vi "Main.vi"(11 "Module Admin":refnum<class "Delacor_lib_QMH_Module Admin.lvclass">) -> ()   [LabVIEW 2024, in "Handheld Scanner.lvlib"]
doc: "This template is based off of the Queued Message Handler design pattern and the Queued Message Handler project template that ships with LabVIEW.\n\nThe main difference is that the queue is private to this module and communication between modules is performed via Broadcast and Request events.\n\nRequest events are wrapped in public API methods and are handled in the Event Handling Loop (EHL) of this VI. Any module can register for Broadcast events sent by this module. The EHL generates messages based on user interface actions.\n\nThe Message Handling Loop (MHL) processes messages generated by the EHL, or by other messages. The messages are string values, so new messages can be added easily to the Message Cases case structure in the MHL. Each message cluster can also provide an optional value for Message Data, which is a variant that can be converted to whatever message-specific data is required.\n_____\nBased on DQMH Dev Tools: Project Template 7.1.0.1503."
uses:
  Handheld Scanner.lvlib
  <vilib>/Delacor/Delacor QMH/Libraries/Module Admin_class/Delacor_lib_QMH_Module Admin.lvclass
  Module Data--cluster.ctl
  <vilib>/Delacor/Delacor QMH/Libraries/Message Queue_class/Delacor_lib_QMH_Message Queue.lvclass/Delacor_lib_QMH_Message Queue.ctl
  Stop Argument--cluster.ctl
  <vilib>/Delacor/Delacor QMH/Libraries/Module Admin_class/Delacor_lib_QMH_Module Admin.lvclass/Delacor_lib_QMH_Module Admin.ctl
  connect Argument--cluster.ctl
  read data Argument--cluster.ctl
  <vilib>/Utility/miscctls.llb/LVPointTypeDef.ctl
  GUI/Controls/HW Modules.ctl
  <vilib>/Delacor/Delacor QMH/Libraries/Message Queue_class/Delacor_lib_QMH_Enqueue Message (Single).vi
  <vilib>/Delacor/Delacor QMH/Libraries/Module Admin_class/Delacor_lib_QMH_Get External Launch.vi
  <vilib>/Delacor/Delacor QMH/Libraries/Message Queue_class/Delacor_lib_QMH_Message Queue.lvclass
  Controller/Controller.lvlib
panel:
  out "error out":errorcluster
  out "Status":string
  in  "Simulate MHL Error":bool
  in  "Simulate EHL Error":bool
  # "Other processes communicate with this Module via its Public API (wrappers for its Request Events).\n\nThis Module communicates with other processes via its Broadcast Events.\nAny process that wants to receive these messages can register for this module's Broadcast events."
  # "This template is for the DQMH framework. See the block diagram for more information on how to use this template."
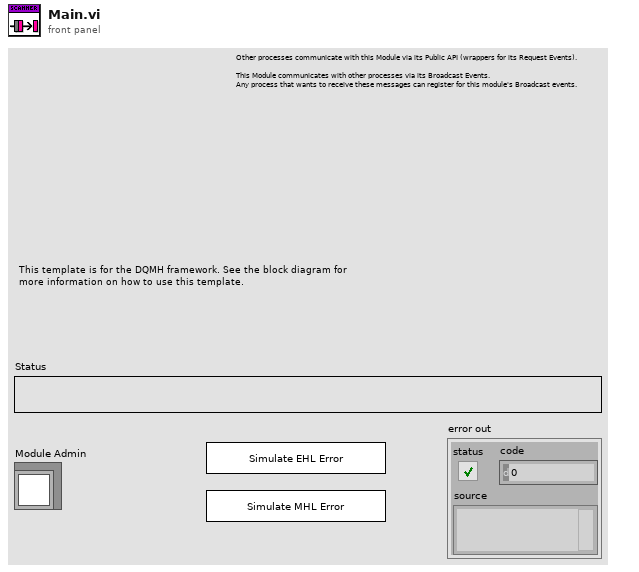
[diagram p1: front panel]
types:
  T1 = typedef "Handheld Scanner.lvlib/Request Events--cluster.ctl" = cluster{"Stop Module":refnum<user-event>, "Show Panel":refnum<user-event>, "Hide Panel":refnum<user-event>, "Get Module Execution Status":refnum<user-event>, "Show Diagram":refnum<user-event>, "connect":refnum<user-event>, "Private.read data":refnum<user-event>}
  T2 = typedef "Handheld Scanner.lvlib/Module Data--cluster.ctl" = cluster{"Status":string}
  T3 = enum32{"invalid lock state", "Not Locked", "Locked (No Password)", "Password-protected"}
  T4 = typedef "Handheld Scanner.lvlib/Stop Argument--cluster.ctl" = cluster{"Origin":string, "Exit via Stop Module Req?":bool, "Wait for Module to stop?":bool}
  T5 = typedef "Handheld Scanner.lvlib/connect Argument--cluster.ctl" = cluster{"VISA":refnum<visa-resource-name>}
  T6 = typedef "Handheld Scanner.lvlib/read data Argument--cluster.ctl" = cluster{"Boolean":bool}
  T7 = typedef "LVPointTypeDef.ctl" = cluster{"Horizontal":i16, "Vertical":i16}
  T8 = enum32{"Invalid", "Standard", "Closed", "Hidden", "Minimized", "Maximized"}
  T9 = typedef "HW Modules.ctl" = string
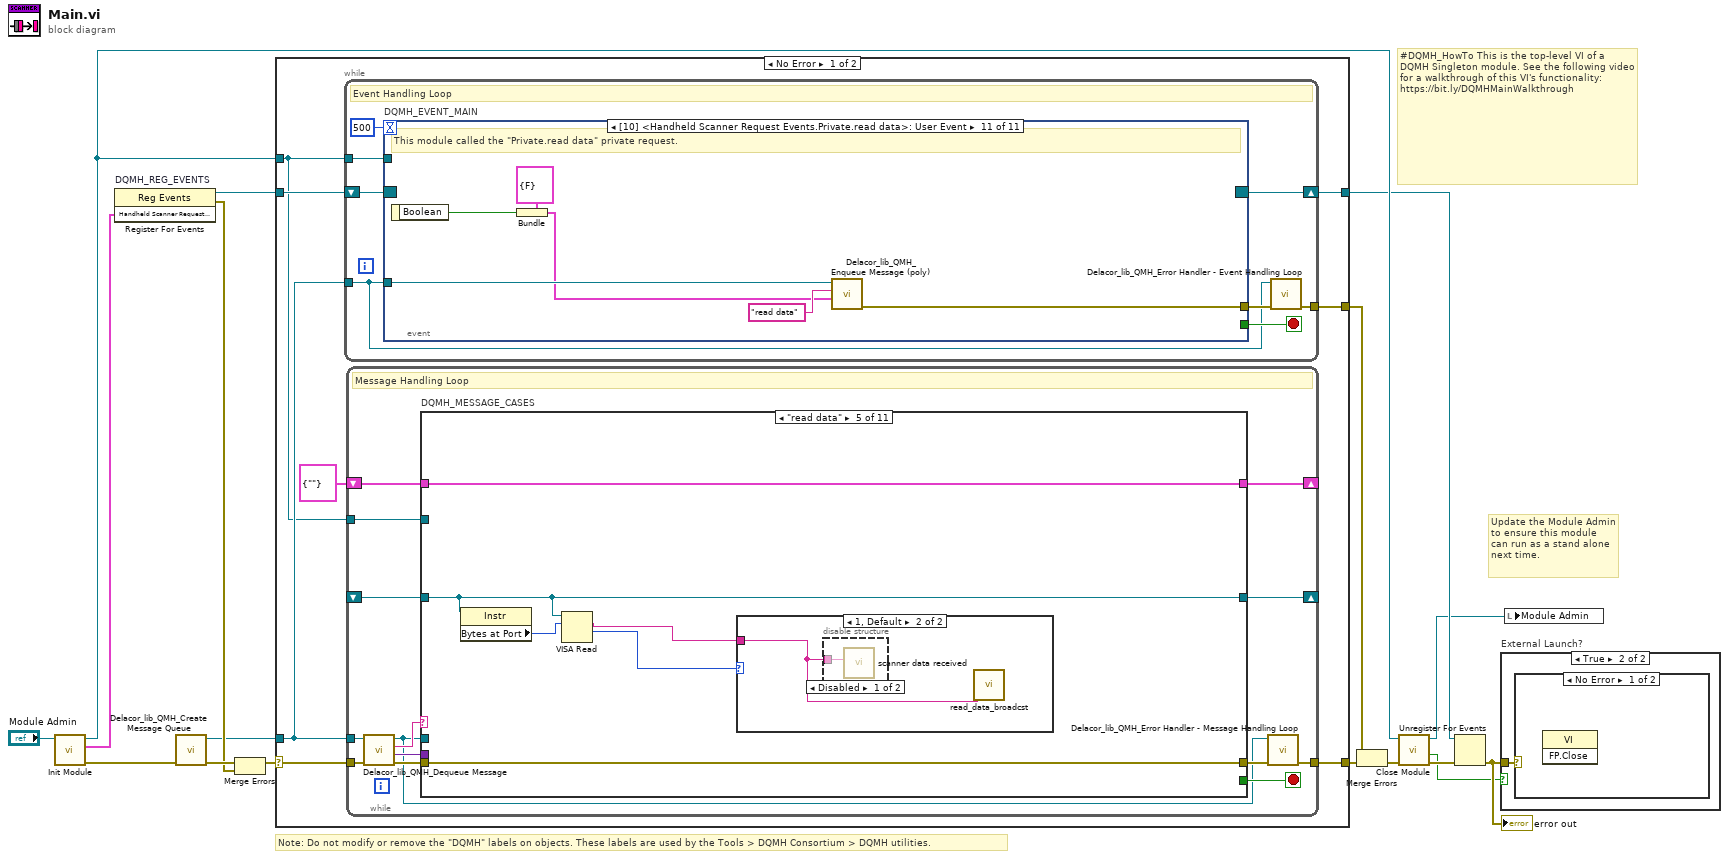
[diagram p0: block diagram]
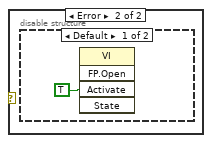
[diagram p3: hidden frame]
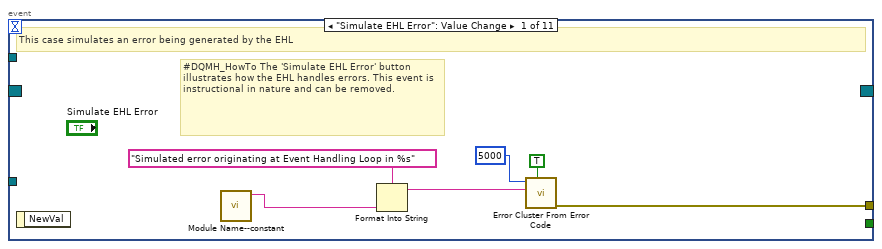
[diagram p5: hidden frame]
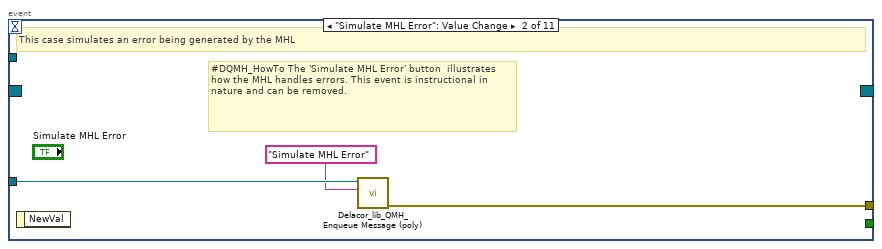
[diagram p6: hidden frame]
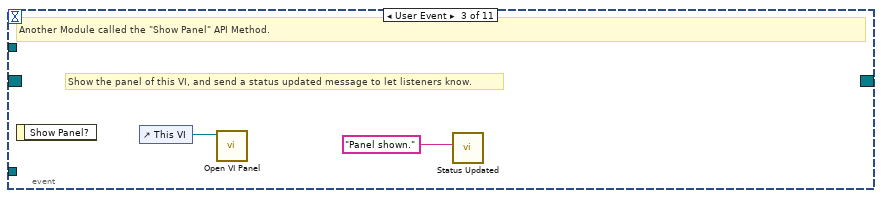
[diagram p7: hidden frame]
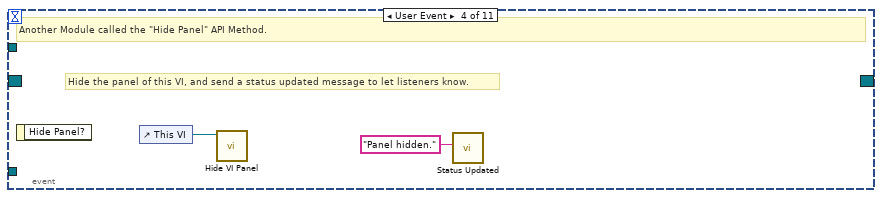
[diagram p8: hidden frame]
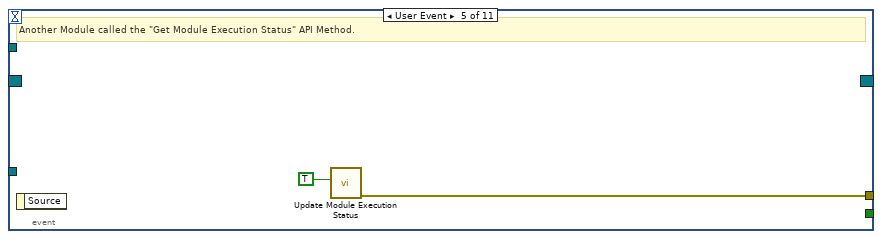
[diagram p9: hidden frame]
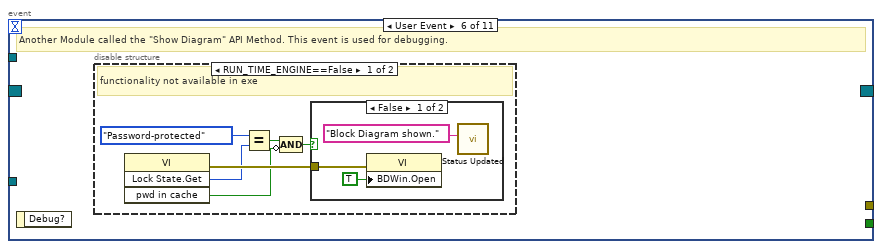
[diagram p10: hidden frame]
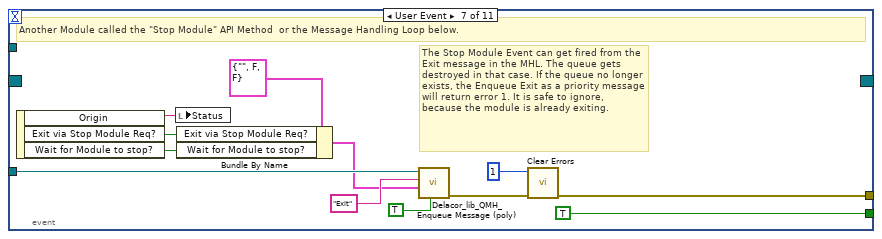
[diagram p13: hidden frame]
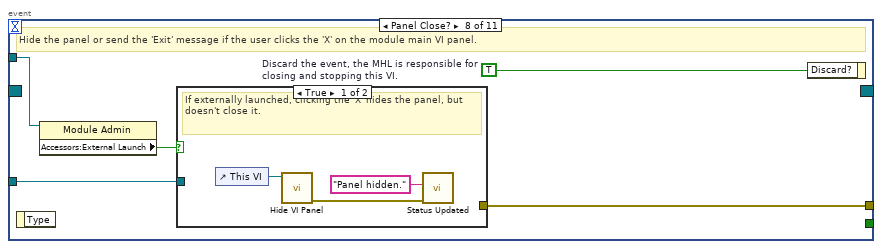
[diagram p14: hidden frame]
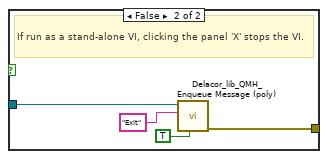
[diagram p15: hidden frame]
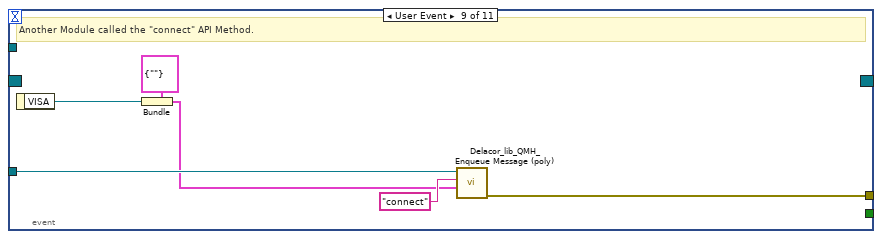
[diagram p16: hidden frame]
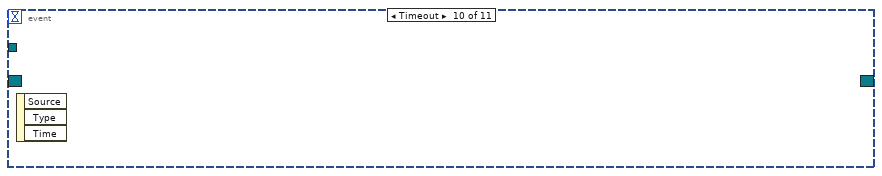
[diagram p17: hidden frame]
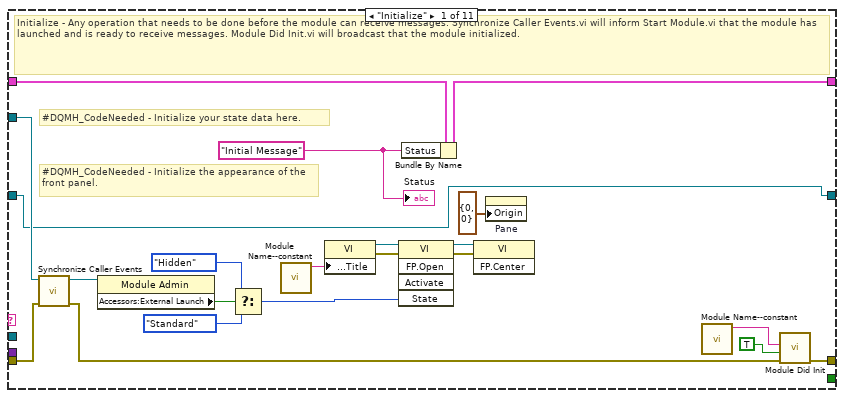
[diagram p18: hidden frame]
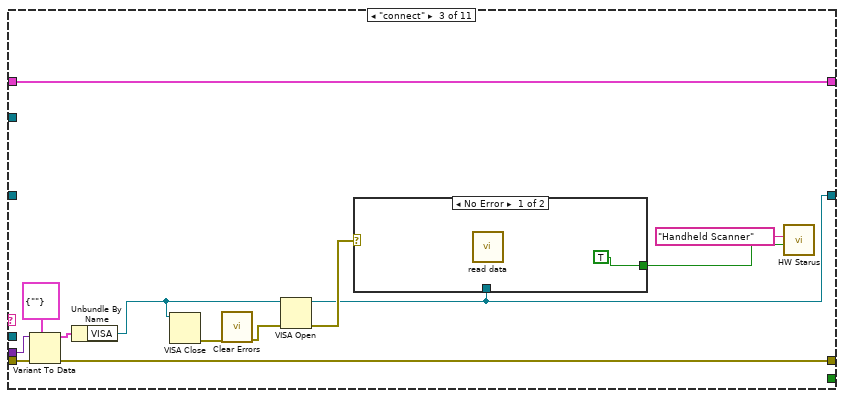
[diagram p20: hidden frame]
diagram:
  # "#DQMH_HowTo This is the top-level VI of a DQMH Singleton module. See the following video for a walkthrough of this VI's functionality: https://bit.ly/DQMHMainWalkthrough"
  # "Note: Do not modify or remove the \"DQMH\" labels on objects. These labels are used by the Tools > DQMH Consortium > DQMH utilities."
  # "Update the Module Admin to ensure this module can run as a stand alone next time."
  n1 = call "Init Module.vi"("Singleton Module Admin in"="Module Admin") -> ("error out"=w16:errorcluster, "Handheld Scanner Request Events"=w5:T1, "Singleton Module Admin out"=w8:refnum<class "Delacor_lib_QMH_Module Admin.lvclass">)  [unwired: 8 in]
  n2 = register-events "DQMH_REG_EVENTS"(w5) -> (reference out=w6:refnum<event-registration>, error out=w9:errorcluster)  [unwired: 2 in]
  n3 = call <vilib>:"Delacor_lib_QMH_Create Message Queue.vi"("error in"=w16) -> ("error out"=w11:errorcluster, "Message Queue"=w4:refnum<class "Delacor_lib_QMH_Message Queue.lvclass">)  [unwired: 9 in]
  n4 = Merge Errors(w11, w9) -> (w10:errorcluster)
  n5 = case shown="No Error" w10 {
    selector: w10 -> [w23 w232]
    tunnel: [w25 w231] -> w17
    tunnel: [w22 w230] -> w7
    tunnel: w6 -> [w20 w230]
    tunnel: w4 -> [w19 w225]
    tunnel: [w24 _] -> w14
    tunnel: w8 -> [w18 w226]
    frame No Error {
      n6 = while {
        tunnel: w19 -> [w27]
        shift-right: [w30] -> w22
        shift-left: w20 -> [w31]
        tunnel: [w32] -> w24
        tunnel: w18 -> [w28]
        stop <- w29 stop-if-true
        # "Event Handling Loop"
        n7 = event "DQMH_EVENT_MAIN" shown="[10] <Handheld Scanner Request Events.Private.read data>: User Event" {
          selector: w31 -> [_ _ _ _ _ _ _ _ _ _ _]
          dyn-events: [_ _ _ _ _ _ _ _ _ _ _] -> w30
          timeout: 500 -> [_ _ _ _ _ _ _ _ _ _ _]
          tunnel: [_ _ _ _ _ _ TRUE ("Discard?") _ _ _ _] -> w29
          tunnel: w27 -> [_ w41 _ _ _ _ w65 w72 w87 _ w93]
          tunnel: [w39 w42 _ _ w48 _ w68 w74 w82 _ w88] -> w33
          tunnel: w28 -> [_ _ _ _ _ _ _ w71 _ _ _]
          event "Simulate EHL Error": Value Change {
            # "#DQMH_HowTo The 'Simulate EHL Error' button  illustrates how the EHL handles errors. This event is instructional in nature and can be removed."
            # "This case simulates an error being generated by the EHL"
            n8 = event-data() -> ()  [unwired: 1 in, 1 out]
            n9 = call "Module Name--constant.vi"() -> ("Module Name"=w36:string)  [unwired: 11 in]
            n10 = Format Into String(format string="Simulated error originating at Event Handling Loop in %s", w36) -> (resulting string=w37:string)  [unwired: 2 in, 1 out]
            n11 = call <vilib>:"Error Cluster From Error Code.vi"("show call chain? (False)"=TRUE, "error message (\"\")"=w37, "error code (0)"=5000) -> ("error out"=w39:errorcluster)  [unwired: 6 in]
          }
          event "Simulate MHL Error": Value Change {
            # "#DQMH_HowTo The 'Simulate MHL Error' button  illustrates how the MHL handles errors. This event is instructional in nature and can be removed."
            # "This case simulates an error being generated by the MHL"
            n12 = event-data() -> ()  [unwired: 1 in, 1 out]
            n13 = call-poly <vilib>:"Delacor_lib_QMH_Enqueue Message (poly).vi"("Message"="Simulate MHL Error", "Message Queue in"=w41) -> ("error out"=w42:errorcluster)  [unwired: 8 in, 1 out]
          }
          event User Event {
            # "Show the panel of this VI, and send a status updated message to let listeners know."
            # "Another Module called the \"Show Panel\" API Method."
            n14 = event-data() -> ()  [unwired: 1 in, 1 out]
            n15 = control-ref of="This VI"() -> (w44:refnum<vi>)
            n16 = call "Open VI Panel.vi"("VI"=w44) -> ()  [unwired: 10 in, 1 out]
            n17 = call "Status Updated.vi"("Status"="Panel shown." ("format string")) -> ()  [unwired: 10 in, 1 out]
          }
          event User Event {
            # "Hide the panel of this VI, and send a status updated message to let listeners know."
            # "Another Module called the \"Hide Panel\" API Method."
            n18 = event-data() -> ()  [unwired: 1 in, 1 out]
            n19 = control-ref of="This VI"() -> (w46:refnum<vi>)
            n20 = call "Hide VI Panel.vi"("VI"=w46) -> ()  [unwired: 10 in, 1 out]
            n21 = call "Status Updated.vi"("Status"="Panel hidden." ("format string")) -> ()  [unwired: 10 in, 1 out]
          }
          event User Event {
            # "Another Module called the \"Get Module Execution Status\" API Method."
            n22 = event-data() -> ()  [unwired: 1 in, 1 out]
            n23 = call "Update Module Execution Status.vi"("Running?"=TRUE) -> ("error out"=w48:errorcluster)  [unwired: 10 in]
          }
          event User Event {
            # "Another Module called the \"Show Diagram\" API Method. This event is used for debugging."
            n24 = event-data() -> ()  [unwired: 1 in, 1 out]
            n25 = disable-structure shown="RUN_TIME_ENGINE==False" {
              frame condition #0 (active) {
                # "functionality not available in exe"
                n26 = invoke on="Invoke Node" class="VI" method="Lock State.Get"() -> (error out=w54:errorcluster, "Get Lock State"=w53:T3, "pwd in cache"=w50:bool)  [unwired: 4 in, 1 out]
                n27 = Equal?(x=T3."Password-protected", y=w53) -> (x = y?=w51:bool)
                n28 = Compound Arithmetic op=AND(w51, invert w50) -> (w49:bool)
                n29 = case shown="False" w49 {
                  tunnel: w54 -> [w57 _]
                  frame False {
                    n30 = property on="Property Node" class="VI"(error in=w57, "BDWin.Open"=TRUE ("Block Diagram Window:Open")) -> ()  [unwired: 1 in, 2 out]
                    n31 = call "Status Updated.vi"("Status"="Block Diagram shown." ("format string")) -> ()  [unwired: 10 in, 1 out]
                  }
                  frame True {
                    # "Password-protected VI, and the password is not in the cache. Do not show the diagram."
                  }
                }
              }
              frame condition #1 {
              }
            }
          }
          event User Event {
            # "The Stop Module Event can get fired from the Exit message in the MHL. The queue gets destroyed in that case. If the queue no longer exists, the Enqueue Exit as a priority message will return error 1. It is safe to ignore, because the module is already exiting."
            # "Another Module called the \"Stop Module\" API Method  or the Message Handling Loop below."
            n32 = event-data() -> ("Origin"=w64:string, "Exit via Stop Module Req?"=w60:bool, "Wait for Module to stop?"=w59:bool)  [unwired: 1 in]
            n33 = local write "Status"(w64) -> ()
            n34 = Bundle By Name(cluster=T4 {"Origin"="", "Exit via Stop Module Req?"=FALSE, "Wait for Module to stop?"=FALSE} ("Stop Argument"), "Exit via Stop Module Req?"=w60, "Wait for Module to stop?"=w59) -> (w58:T4)
            n35 = call-poly <vilib>:"Delacor_lib_QMH_Enqueue Message (poly).vi"("Priority Message? (F)"=TRUE, "Message Data"=w58, "Message"="Exit", "Message Queue in"=w65) -> ("error out"=w69:errorcluster)  [unwired: 6 in, 1 out]
            n36 = call <vilib>:"Clear Errors.vi"("error in (no error)"=w69, "specific error code to clear (0: all)"=1) -> ("error out"=w68:errorcluster)  [unwired: 4 in, 1 out]
          }
          event Panel Close? {
            w73 = TRUE  # Discard the event, the MHL is responsible for closing and stopping this VI.
            # "Hide the panel or send the 'Exit' message if the user clicks the 'X' on the module main VI panel."
            n37 = event-data() -> ()  [unwired: 1 in, 1 out]
            n38 = property on="Property Node" class="Module Admin"(reference=w71) -> ("Accessors:External Launch"=w70:bool)  [unwired: 1 in, 2 out]
            n39 = case shown="True" w70 {
              tunnel: w72 -> [_ w80]
              tunnel: [_ w81] -> w74
              frame True {
                # "If externally launched, clicking the 'X' hides the panel, but doesn't close it."
                n40 = control-ref of="This VI"() -> (w77:refnum<vi>)
                n41 = call "Hide VI Panel.vi"("VI"=w77) -> ("error out"=w75:errorcluster)  [unwired: 10 in]
                n42 = call "Status Updated.vi"("error in"=w75, "Status"="Panel hidden." ("format string")) -> ()  [unwired: 9 in, 1 out]
              }
              frame False {
                # "If run as a stand-alone VI, clicking the panel 'X' stops the VI."
                n43 = call-poly <vilib>:"Delacor_lib_QMH_Enqueue Message (poly).vi"("Priority Message? (F)"=TRUE, "Message"="Exit", "Message Queue in"=w80) -> ("error out"=w81:errorcluster)  [unwired: 7 in, 1 out]
              }
            }
            n44 = event-data ("Event Filter Node")("Discard?"=w73) -> ()  [unwired: 1 in, 1 out]
          }
          event User Event {
            # "Another Module called the \"connect\" API Method."
            n45 = event-data() -> ("VISA"=w83:refnum<visa-resource-name>)  [unwired: 1 in]
            n46 = Bundle(cluster=T5 {"VISA"=""} ("connect Argument"), "VISA"=w83) -> (w84:T5)
            n47 = call-poly <vilib>:"Delacor_lib_QMH_Enqueue Message (poly).vi"("Message Data"=w84, "Message"="connect", "Message Queue in"=w87) -> ("error out"=w82:errorcluster)  [unwired: 7 in, 1 out]
          }
          event Timeout {
            n48 = event-data() -> ()  [unwired: 1 in, 3 out]
          }
          event User Event {
            # "This module called the \"Private.read data\" private request."
            n49 = event-data() -> ("Boolean"=w89:bool)  [unwired: 1 in]
            n50 = Bundle(cluster=T6 {"Boolean"=FALSE} ("read data Argument"), "Boolean"=w89) -> (w90:T6)
            n51 = call-poly <vilib>:"Delacor_lib_QMH_Enqueue Message (poly).vi"("Message Data"=w90, "Message"="read data", "Message Queue in"=w93) -> ("error out"=w88:errorcluster)  [unwired: 7 in, 1 out]
          }
        }
        n52 = call-dynamic "Delacor_lib_QMH_Error Handler - Event Handling Loop.vi"("error in"=w33, "Message Queue in"=w27) -> ("dup error in"=w32:errorcluster)  [unwired: 8 in, 1 out]
      }
      n53 = while {
        tunnel: w19 -> [w96]
        shift-right: [w104] -> _
        shift-left: T2 {"Status"=""} ("Data Cluster") -> [w105]
        tunnel: w23 -> [w107]
        tunnel: [w99] -> w25
        tunnel: w18 -> [w100]
        shift-right: [w95] -> _
        shift-left: _ -> [w94]
        stop <- w103 stop-if-true
        # "Message Handling Loop"
        n54 = call-dynamic "Delacor_lib_QMH_Dequeue Message.vi"("error in"=w107, "Message Queue in"=w96) -> ("error out"=w106:errorcluster, "Message Data"=w101:variant, "Message"=w102:string, "Message Queue out"=w97:refnum<class "Delacor_lib_QMH_Message Queue.lvclass">)  [unwired: 6 in]
        n55 = case "DQMH_MESSAGE_CASES" shown="\"read data\"" w102 {
          selector: w102 -> [_ _ _ _ _ _ _ _ _ _ w220]
          tunnel: w97 -> [_ _ _ _ _ _ _ _ w184 w207 _]
          tunnel: w106 -> [w126 w131 w144 w154 w160 w166 w169 w179 w191 w213 w223]
          tunnel: [w124 w131 w142 w151 w160 w165 w169 w178 w187 w208 w224] -> w98
          tunnel: w105 -> [w115 w130 w143 w153 w159 w164 w168 w176 w186 w206 w221]
          tunnel: [w114 w130 w143 w153 w159 w164 w168 w176 w186 w206 w221] -> w104
          tunnel: [_ _ _ _ _ _ _ _ _ w205 _] -> w103
          tunnel: w101 -> [_ _ w141 w150 _ _ _ _ w185 w204 _]
          tunnel: w100 -> [w116 _ _ _ _ _ _ _ w183 w199 _]
          tunnel: [w108 w129 w135 w152 w156 w163 w167 w170 w180 w198 w214] -> w95
          tunnel: w94 -> [w108 w129 _ w152 w156 w163 w167 w170 w180 w198 w214]
          frame "Initialize" {
            w110 = "Initial Message" ("Initial Message")
            # "#DQMH_CodeNeeded - Initialize the appearance of the front panel."
            # "#DQMH_CodeNeeded - Initialize your state data here."
            # "Initialize - Any operation that needs to be done before the module can receive messages. Synchronize Caller Events.vi will inform Start Module.vi that the module has launched and is ready to receive messages. Module Did Init.vi will broadcast that the module initialized."
            n56 = call "Synchronize Caller Events.vi"("error in"=w126, "Singleton Module Admin in"=w116) -> ("error out"=w125:errorcluster, "Singleton Module Admin out"=w111:refnum<class "Delacor_lib_QMH_Module Admin.lvclass">)  [unwired: 8 in]
            n57 = property on="Property Node" class="Module Admin"(reference=w111) -> ("Accessors:External Launch"=w120:bool)  [unwired: 1 in, 2 out]
            n58 = Select(t=T8."Hidden" ("State"), s=w120, f=T8."Standard" ("State")) -> (s? t:f=w117:T8)
            n59 = call "Module Name--constant.vi"() -> ("Module Name"=w123:string)  [unwired: 11 in]
            n60 = property on="Property Node" class="VI"("Front Panel.Title"=w123) -> (reference out=w122:refnum<vi>, error out=w128:errorcluster)  [unwired: 2 in]
            n61 = invoke on="Invoke Node" class="VI" method="FP.Open"(reference=w122, error in=w128, "State"=w117) -> (reference out=w121:refnum<vi>, error out=w127:errorcluster)  [unwired: 2 in, 3 out]
            n62 = Bundle By Name(cluster=w115, "Status"=w110) -> (w114:T2)
            n63 = invoke on="Invoke Node" class="VI" method="FP.Center"(reference=w121, error in=w127) -> ()  [unwired: 1 in, 3 out]
            n64 = property on="Pane" class="Pane"("Origin"=T7 {"Horizontal"=0, "Vertical"=0}) -> ()  [unwired: 2 in, 2 out]
            n65 = call "Module Name--constant.vi"() -> ("Module Name"=w112:string)  [unwired: 11 in]
            n66 = call "Module Did Init.vi"("error in"=w125, "Initialized?"=TRUE, "Origin"=w112) -> ("error out"=w124:errorcluster)  [unwired: 8 in]
            "Status" <- w110
          }
          frame "---Module Specific---" {
            # "Separator -- The following cases handle messages specific to this Module."
          }
          frame "connect" {
            n67 = Variant To Data(error in=w144, type=T5 {"VISA"=""} ("connect Argument"), Variant=w141) -> (data=w139:T5, error out=w142:errorcluster)
            n68 = Unbundle By Name(w139) -> ("VISA"=w134:refnum<visa-resource-name>)
            n69 = VISA Close(VISA resource name=w134) -> (error out=w133:errorcluster)  [unwired: 1 in]
            n70 = call <vilib>:"Clear Errors.vi"("error in (no error)"=w133) -> ("error out"=w132:errorcluster)  [unwired: 5 in, 1 out]
            n71 = VISA Open(error in (no error)=w132, VISA resource name=w134) -> (VISA resource name=w135:refnum<visa-resource-name>, error out=w138:errorcluster)  [unwired: 3 in]
            n72 = case shown="No Error" w138 {
              tunnel: [TRUE FALSE] -> w136
              tunnel: w135 -> [_ w146]
              frame No Error {
                n73 = call "read data.vi"() -> ()  [unwired: 11 in, 1 out]
              }
              frame Error {
                n74 = call "connect.vi"("VISA"=w146) -> ()  [unwired: 10 in, 1 out]
              }
            }
            n75 = call "HW Starus.vi"("Status"=w136, "HW Module"=T9 "Handheld Scanner") -> ()  [unwired: 9 in, 1 out]
          }
          frame "Read" {
            # "#DQMH_CodeNeeded\n1. Configure this Message Case for handling the \"read data\" message.\n2. Delete or edit this label when done."
            n76 = Variant To Data(error in=w154, type=T6 {"Boolean"=FALSE} ("read data Argument"), Variant=w150) -> (data=w148:T6, error out=w151:errorcluster)
            n77 = Unbundle By Name(w148) -> ()  [unwired: 1 out]
          }
          frame "read data" {
            n78 = property class="Instr"(reference=w156) -> ("Bytes at Port"=w155:u32)  [unwired: 1 in, 2 out]
            n79 = VISA Read(VISA resource name=w156, byte count=w155) -> (read buffer=w157:string, return count=w158:u32)  [unwired: 1 in, 2 out]
            n80 = case shown="1, Default" w158 {
              tunnel: w157 -> [_ w161]
              frame 0 {
              }
              frame 1, Default {
                n81 = disable-structure shown="Disabled" {
                  disable-tunnel: w161 -> [w162 _]
                  frame Disabled {
                    n82 = call "scanner data received.vi"("scanner read"=w162) -> ()  [unwired: 10 in, 1 out]
                  }
                  frame Enabled {
                  }
                }
                n83 = call "read_data_broadcst.vi"("data read"=w161) -> ()  [unwired: 10 in, 1 out]
              }
            }
          }
          frame "---Copy This Frame---" {
            # "Duplicate this frame when creating new messages.  Change this comment in the duplicated frame to describe this message."
            n84 = Merge Errors(w166) -> (w165:errorcluster)
          }
          frame "---Exit and Error Handling---" {
            # "Separator - The following cases handle errors and exit messages."
          }
          frame "Simulate MHL Error" {
            # "#DQMH_HowTo The 'Simulate MHL Error' button  illustrates how the MHL handles errors. This event is instructional in nature and can be removed."
            # "Simulate an error occurring at the MHL"
            n85 = call "Module Name--constant.vi"() -> ("Module Name"=w172:string)  [unwired: 11 in]
            n86 = Format Into String(format string="Simulated error originating at Message Handling Loop in %s", w172) -> (resulting string=w173:string)  [unwired: 2 in, 1 out]
            n87 = call <vilib>:"Error Cluster From Error Code.vi"("show call chain? (False)"=TRUE, "error message (\"\")"=w173, "error code (0)"=5001) -> ("error out"=w177:errorcluster)  [unwired: 6 in]
            n88 = Merge Errors(w179, w177) -> (w178:errorcluster)
          }
          frame "Error" {
            # "#DQMH_CodeRecommended - If the module is running in standalone mode (External Launch = FALSE), this code will pop up an error dialog and call the 'Exit' message if an error occurs. Add more fine-grained error management here."
            # "Error - Check the error message data and respond accordingly. This message is sent by the \"Error Handler\" VIs at the end of each loop in this application."
            n89 = property on="Property Node" class="Module Admin"(reference=w183) -> ("Accessors:External Launch"=w182:bool)  [unwired: 1 in, 2 out]
            n90 = Variant To Data(error in=w191, type=errorcluster {"status"=FALSE, "code"=0, "source"=""} ("error constant"), Variant=w185) -> (data=w181:errorcluster, error out=w189:errorcluster)
            n91 = local write "error out"(w181) -> ()
            n92 = call "Error Reported.vi"("Error"=w181) -> ()  [unwired: 10 in, 1 out]
            n93 = case shown="False" w182 {
              tunnel: [w196 _] -> w188
              tunnel: w184 -> [w194 _]
              tunnel: w181 -> [w195 _]
              frame False {
                n94 = disable-structure shown="Default" {
                  disable-tunnel: w195 -> [w197 _]
                  frame condition #0 (active) {
                    # "If the module is running standalone, then pop up an error dialog and call the \"Exit\" message."
                    n95 = call <vilib>:"Simple Error Handler.vi"("error in (no error)"=w197) -> ()  [unwired: 4 in, 5 out]
                  }
                  frame condition #1 {
                    # "To prevent the Simple Error Handler VI from being loaded (e.g. when deploying to a Real-Time target), add the Conditional Disable Symbol \"DQMH_Disable_SEH\" to your project and set it to TRUE."
                  }
                }
                n96 = call-poly <vilib>:"Delacor_lib_QMH_Enqueue Message (poly).vi"("Priority Message? (F)"=TRUE, "Message"="Exit", "Message Queue in"=w194) -> ("error out"=w196:errorcluster)  [unwired: 7 in, 1 out]
              }
              frame True {
                # "If the module was launched externally, calling the Error Reported broadcast VI is the only action performed by the \"Error\" message. The module's caller can then process the error appropriately."
              }
            }
            n97 = Merge Errors(w189, w188) -> (w187:errorcluster)
          }
          frame "Exit" {
            w203 = 91  # 91: not all Exit messages will have an argument
            w205 = TRUE  # Stop the VI
            # "Release the message queue reference"
            # "#DQMH_CodeNeeded - Add any required cleanup code here."
            # "Exit - Exit the application."
            n98 = Variant To Data(error in=w213, type=T4 {"Origin"="", "Exit via Stop Module Req?"=FALSE, "Wait for Module to stop?"=FALSE} ("Stop Argument"), Variant=w204) -> (data=w201:T4, error out=w210:errorcluster)
            n99 = call <vilib>:"Clear Errors.vi"("error in (no error)"=w210, "specific error code to clear (0: all)"=w203) -> ("error out"=w212:errorcluster)  [unwired: 4 in, 1 out]
            n100 = control-ref of="This VI"() -> (w200:refnum<vi>)
            n101 = call-dynamic "Delacor_lib_QMH_Release Message Queue.vi"("error in"=w212, "Message Queue"=w207) -> ("error out"=w211:errorcluster)  [unwired: 9 in]
            n102 = call "Handle Exit.vi"("Stop Argument"=w201, "Admin in"=w199, "VI reference"=w200) -> ("error out"=w209:errorcluster)  [unwired: 7 in, 1 out]
            n103 = Merge Errors(w211, w209) -> (w208:errorcluster)
            n104 = call "Error Reported.vi"("Error"=w208) -> ()  [unwired: 10 in, 1 out]
          }
          frame Default {
            # "'Default' case only runs if there is a message that isn't defined in any of the other cases.  Output a programming error."
            n105 = call "Module Name--constant.vi"() -> ("Module Name"=w219:string)  [unwired: 11 in]
            n106 = Format Into String(format string="The invalid message string \"%s\" was received in the Message Handling Loop for module \"%s\".", w220, w219) -> (resulting string=w215:string)  [unwired: 2 in, 1 out]
            n107 = call <vilib>:"Error Cluster From Error Code.vi"("show call chain? (False)"=TRUE, "error message (\"\")"=w215, "error code (0)"=1) -> ("error out"=w222:errorcluster)  [unwired: 6 in]
            n108 = Merge Errors(w223, w222) -> (w224:errorcluster)
          }
        }
        n109 = call-dynamic "Delacor_lib_QMH_Error Handler - Message Handling Loop.vi"("error in"=w98, "Message Queue in"=w97) -> ("dup error in"=w99:errorcluster)  [unwired: 8 in, 1 out]
      }
    }
    frame Error {
      # "Synchronize Caller Events.vi will inform Start Module.vi that the module has launched and will let the code calling Start Module.vi register for broadcasts and would permit the caller receive the broadcast that an error occurred at launch time."
      n110 = call-dynamic "Delacor_lib_QMH_Release Message Queue.vi"("error in"=w232, "Message Queue"=w225) -> ("error out"=w231:errorcluster)  [unwired: 9 in]
      n111 = call "Synchronize Caller Events.vi"("Singleton Module Admin in"=w226) -> ("error out"=w233:errorcluster)  [unwired: 9 in, 1 out]
      n112 = call "Module Name--constant.vi"() -> ("Module Name"=w229:string)  [unwired: 11 in]
      n113 = Format Into String(format string="An error occurred during initialization. %s is no longer running.", w229) -> (resulting string=w227:string)  [unwired: 2 in, 1 out]
      n114 = Merge Errors(w231, w233) -> (w234:errorcluster)
      n115 = call "Error Reported.vi"("Additional Information"=w227, "Error"=w234) -> ()  [unwired: 9 in, 1 out]
    }
  }
  n116 = Merge Errors(w14, w17) -> (w13:errorcluster)
  n117 = call "Close Module.vi"("error in"=w13, "Module Admin in"=w8) -> ("error out"=w15:errorcluster, "External Launch"=w1:bool, "Module Admin out"=w2:refnum<class "Delacor_lib_QMH_Module Admin.lvclass">)  [unwired: 7 in]
  n118 = Unregister For Events(event registration refnum=w7, error in=w15) -> (error out=w12:errorcluster)
  "error out" <- w12
  n119 = case "External Launch?" shown="True" w1 {
    tunnel: w12 -> [_ w235]
    frame False {
    }
    frame True {
      n120 = case shown="No Error" w235 {
        frame No Error {
          n121 = invoke on="Invoke Node" class="VI" method="FP.Close"() -> ()  [unwired: 3 in, 3 out]
        }
        frame Error {
          n122 = disable-structure shown="Default" {
            frame condition #0 (active) {
              n123 = invoke class="VI" method="FP.Open"("Activate"=TRUE ("Activate?")) -> ()  [unwired: 4 in, 5 out]
            }
            frame condition #1 {
              # "Don't show panel on error if running inside a built EXE."
            }
          }
        }
      }
    }
  }
  n124 = local write "Module Admin"(w2) -> ()
